vi "PhotonVision_Globals.vi"() -> ()   [LabVIEW 2019, in "PhotonVisionLib.lvlib"]
uses:
  PhotonVisionLib.lvlib
panel:
  out "PV_TimeSyncServRcvIP":u32
  out "PV_TimeSyncClientLastRcvId":i8
  out "PV_TimeSyncClientLastRcvVer":i8
  out "PV_TimeSyncClientReadErr":bool
  out "PV_TimeSyncClientWriteErr":bool
  out "PV_TimeSyncServReadErr":bool
  out "PV_TimeSyncServWriteErr":bool
  out "PV_TimeSyncClientTimeOffset":i64
  out "PV_TimeSyncClientLastRcvTime":i64
  out "PV_TimeSyncClientLoopCnt":i32
  out "PV_TimeSyncClientLastSentTime":i64
  out "PV_TimeSyncClientStop":bool
  out "PV_TimeSyncServLoopCount":i32
  out "PV_TimeSyncServStop":bool
  out "PV_TimeSyncServLastSentTime":i64
  out "PV_TimeSyncServLastRcvTim":i64
  out "PV_TimeSyncServLastRcvId":i8
  out "PV_TimeSyncServLastRcvVer":i8
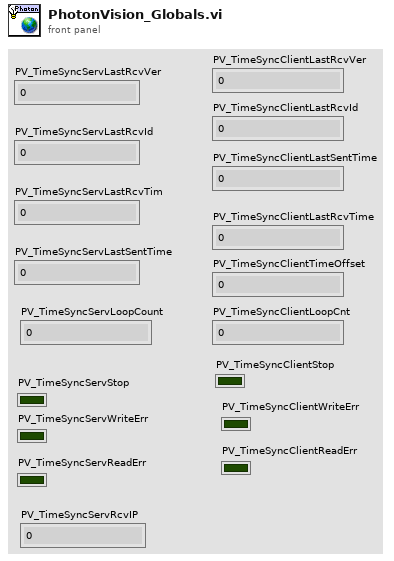
[diagram p1: front panel]
diagram:
